vi "NI VeriStand - Get Parameter Value.vi"   [LabVIEW 2020, in "NI_VS ModelManager ExecutionAPI.lvlib"]
doc: "Returns values of model parameters present on the target. You must manually select the polymorphic instance to use."
uses:
  <vilib>/NI VeriStand/Execution/ModelManager/NI_VS ModelManager ExecutionAPI.lvlib
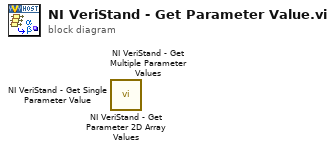
[diagram p0: block diagram]
diagram:
  n1 = call <vilib>:"NI VeriStand - Get Parameter 2D Array Values.vi"() -> ()  [unwired: 9 in, 3 out]
  n2 = call <vilib>:"NI VeriStand - Get Multiple Parameter Values.vi"() -> ()  [unwired: 9 in, 3 out]
  n3 = call <vilib>:"NI VeriStand - Get Single Parameter Value.vi"() -> ()  [unwired: 9 in, 3 out]
